vi "Compute Distance.vi"(8 "Y Image Resolution":i32=240, 9 "X Image Resolution":i32=320, 10 "Particle Scores":T1={"Position"={"Left"=20.0, "Top"=105.0, "Right"=137.0, "Bottom"=145.0}, "Scores"=[95.44871794871796, 94.87179487179486, 82.5, 89.68123807662933, 65.478142885056], "Equiv Size"={"Long"=109.62747244486255, "Short"=40.74708556513232}}) -> (1 "Center Target":bool=TRUE, 2 "Target Angles":cluster{"X":dbl, "Y":dbl}={"X"=-0.0, "Y"=0.0}, 3 "Distance (ft)":dbl=inf)   [LabVIEW 2013]
doc: "Using the camera lens information and the real world size of the target, use trig and simple math to determine the distance to the target. Also returns the location relative to the image center in a (-1 , 1) coordinate system that may be useful for steering the robot."
panel:
  in  "Camera View Angles":cluster{"X":dbl, "Y":dbl}={"X"=54.0, "Y"=40.5}
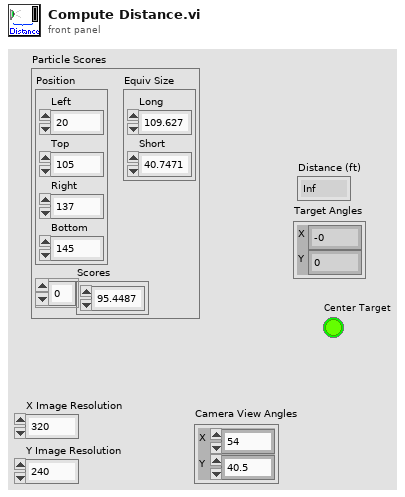
[diagram p1: front panel]
types:
  T1 = cluster{"Position":cluster{"Left":dbl, "Top":dbl, "Right":dbl, "Bottom":dbl}, "Scores":dbl[], "Equiv Size":cluster{"Long":dbl, "Short":dbl}}
  T2 = cluster{"X Image Resolution":i32, "Y Image Resolution":i32}
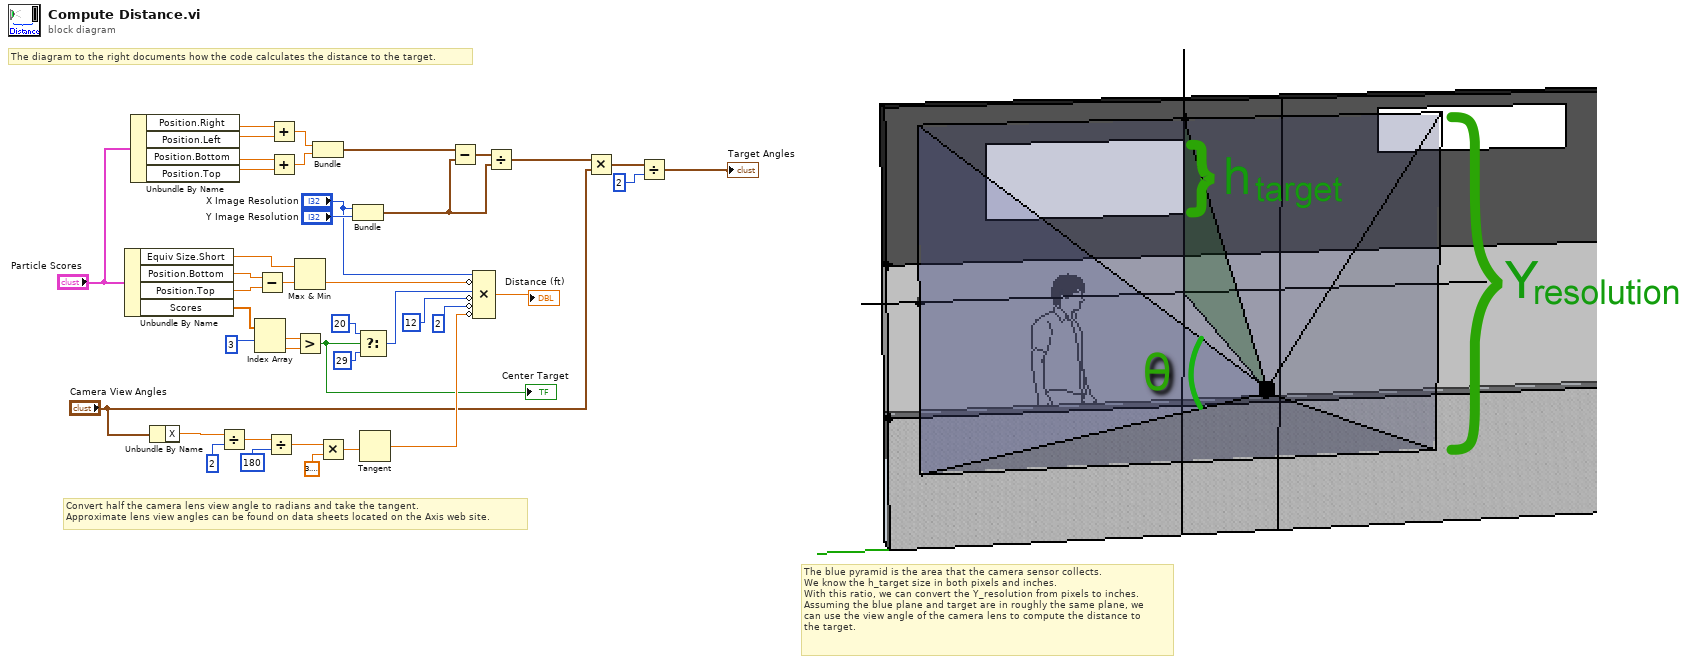
[diagram p0: block diagram]
diagram:
  # "The blue pyramid is the area that the camera sensor collects.\nWe know the h_target size in both pixels and inches.\nWith this ratio, we can convert the Y_resolution from pixels to inches.\nAssuming the blue plane and target are in roughly the same plane, we\ncan use the view angle of the camera lens to compute the distance to\nthe target."
  # "Convert half the camera lens view angle to radians and take the tangent.\nApproximate lens view angles can be found on data sheets located on the Axis web site."
  # "The diagram to the right documents how the code calculates the distance to the target."
  n1 = Unbundle By Name("Particle Scores") -> ("Equiv Size.Short"=w12:dbl, "Position.Bottom"=w35:dbl, "Position.Top"=w34:dbl, "Scores"=w25:dbl[])
  n2 = Unbundle By Name("Particle Scores") -> ("Position.Right"=w29:dbl, "Position.Left"=w30:dbl, "Position.Bottom"=w32:dbl, "Position.Top"=w31:dbl)
  n3 = Unbundle By Name("Camera View Angles") -> ("X"=w4:dbl)
  n4 = Divide(x=w4, y=2) -> (x/y=w38:dbl)
  n5 = Index Array(array=w25, index #1=3) -> (element #1=w14:dbl, element #2=w23:dbl)  [unwired: 1 in]
  n6 = Subtract(x=w35, y=w34) -> (x-y=w11:dbl)
  n7 = Divide(x=w38, y=180) -> (x/y=w37:dbl)
  n8 = Add(x=w29, y=w30) -> (x+y=w28:dbl)
  n9 = Add(x=w32, y=w31) -> (x+y=w27:dbl)
  n10 = Max & Min(x=w12, y=w11) -> (min(x,y)=w10:dbl)  [unwired: 1 out]
  n11 = Greater?(x=w14, y=w23) -> (0:w15:bool)
  "Center Target" <- w15
  n12 = Bundle(w28, w27) -> (w7:cluster{dbl, dbl})  [unwired: 1 in]
  n13 = Multiply(x=w37, y=3.141592653589793) -> (x*y=w39:dbl)
  n14 = Bundle("X Image Resolution"="X Image Resolution", "Y Image Resolution"="Y Image Resolution") -> (w8:T2)  [unwired: 1 in]
  n15 = Select(t=20 ("Target Height (in)"), s=w15, f=29 ("Target Height (in)")) -> (s? t:f=w20:i32)
  n16 = Tangent(1:w39) -> (0:w18:dbl)
  n17 = Subtract(x=w7, y=w8) -> (x-y=w26:cluster{dbl, dbl})
  n18 = Compound Arithmetic op=MULTIPLY("X Image Resolution", invert w10, w20, invert 12, invert 2, invert w18) -> (→"Distance (ft)":dbl)
  n19 = Divide(x=w26, y=w8) -> (x/y=w2:cluster{dbl, dbl})
  n20 = Multiply(x=w2, y="Camera View Angles") -> (x*y=w1:cluster{dbl, dbl})
  n21 = Divide(x=w1, y=2) -> (x/y=→"Target Angles":cluster{dbl, dbl})
